vi "Find Objects (SubVI).vi"(0 "Pixel Data":bool, 1 "Image Width":u16, 2 "Image Height":u16, 9 "Pixel Valid":bool) -> (4 "Particle Statistics":T1, 6 "Output Valid":bool, 10 "End Of Image":bool)   [LabVIEW 2015]
uses:
  <vilib>/visionFPGA/Analysis/ParticleAnalysisReport/SubVIs/WithoutHoles/Particle Statistics without Holes.ctl
  <vilib>/visionFPGA/Controls/IMAQ FPGA Pixel Bus u1x1.ctl
  <vilib>/visionFPGA/Analysis/ParticleAnalysisReport/IMAQ FPGA Particle Analysis Report U1x1.vi
  <vilib>/visionFPGA/NI_VDM_FPGA.lvlib
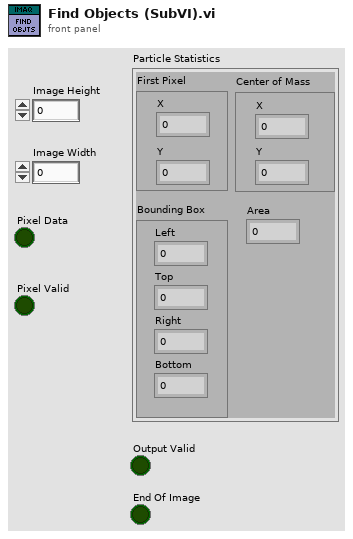
[diagram p1: front panel]
types:
  T1 = typedef "Particle Statistics without Holes.ctl" = cluster{"First Pixel":cluster{"X":i32, "Y":i32}, "Bounding Box":cluster{"Left":i32, "Top":i32, "Right":i32, "Bottom":i32}, "Center of Mass":cluster{"X":fxp<+/-,48,32>, "Y":fxp<+/-,48,32>}, "Area":u32}
  T2 = typedef "IMAQ FPGA Pixel Bus u1x1.ctl" = cluster{"Pixel Data":bool, "DV":bool, "EOL":bool, "EOI":bool, "Data Type":enum16{"U1 x 1"}}
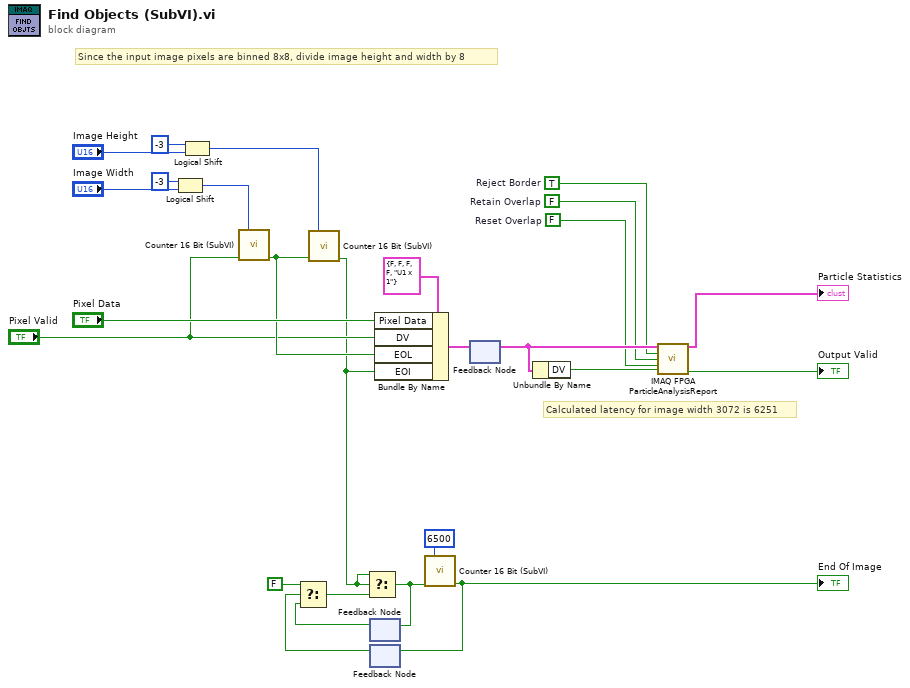
[diagram p0: block diagram]
diagram:
  w10 = FALSE  # Reset Overlap
  w11 = FALSE  # Retain Overlap
  w12 = TRUE  # Reject Border
  # "Calculated latency for image width 3072 is 6251"
  # "Since the input image pixels are binned 8x8, divide image height and width by 8"
  n1 = Logical Shift(y=i16 -3, x="Image Width") -> (x << y=w17:u16)
  n2 = Logical Shift(y=i16 -3, x="Image Height") -> (x << y=w16:u16)
  n3 = call "Counter 16 Bit (SubVI).vi"("Max. Count"=w17, "Enable"="Pixel Valid") -> ("Count End?"=w14:bool)  [unwired: 11 in, 2 out]
  n4 = call "Counter 16 Bit (SubVI).vi"("Max. Count"=w16, "Enable"=w14) -> ("Count End?"=w5:bool)  [unwired: 11 in, 2 out]
  n5 = feedback #1() -> (w4:bool)  [unwired: 1 in]
  n6 = feedback #2() -> (w8:bool)  [unwired: 1 in]
  n7 = Select(t=FALSE, s=w8, f=w4) -> (s? t:f=w3:bool)
  n8 = Select(t=w5, s=w5, f=w3) -> (s? t:f=w6:bool)
  n9 = feedback-in #1(w6) -> ()
  n10 = Bundle By Name(cluster=T2 {"Pixel Data"=FALSE, "DV"=FALSE, "EOL"=FALSE, "EOI"=FALSE, "Data Type"=enum."U1 x 1"} ("Pixel Bus In"), "Pixel Data"="Pixel Data", "DV"="Pixel Valid", "EOL"=w14, "EOI"=w5) -> (w23:T2)
  n11 = call "Counter 16 Bit (SubVI).vi"("Max. Count"=u16 6500, "Enable"=w6) -> ("Count End?"=w2:bool)  [unwired: 11 in, 2 out]
  "End Of Image" <- w2
  n12 = feedback-in #2(w2) -> ()
  n13 = feedback #3() -> (w26:T2)  [unwired: 1 in]
  n14 = feedback-in #3(w23) -> ()
  n15 = Unbundle By Name(w26) -> ("DV"=w24:bool)
  n16 = call-poly <vilib>:"IMAQ FPGA ParticleAnalysisReport.vi"("Pixel Bus In"=w26, "Reject Border"=w12, "Retain Overlap"=w11, "Reset Overlap"=w10, "Input Valid"=w24) -> ("Particle Statistics Out"=→"Particle Statistics":T1, "Output Valid"=→"Output Valid":bool)  [unwired: 7 in, 2 out]
